vi "Valid units Read.vi"(4 "error in (no error)":errorcluster, 6 "Container State":T3, 7 "Display State In":T2) -> (0 "error out":errorcluster, 2 "Value":T1[](array[typedef]), 3 "Display State Out":T2)   [LabVIEW 2015, in "Level (G3).xctl"]
uses:
  Level (G3).xctl
  <vilib>/_xctls/Container State.ctl
  State.ctl
  Utility VIs/Controls/KRing/KRing.xctl
  Utility VIs/Controls/KNumeric (DBL)/KNumeric (DBL).xctl
  Level Units (G3).ctl
  <vilib>/_xctls/XControlSupport.lvlib
panel:
  # "Replace the Value Indicator below with an Indicator of desired type.\nDo not remove this Indicator or the others from the connector pane. \nDo not change the connector pane pattern.\nThe Value Indicator should always be the second terminal from top on the output side in the connector pane."
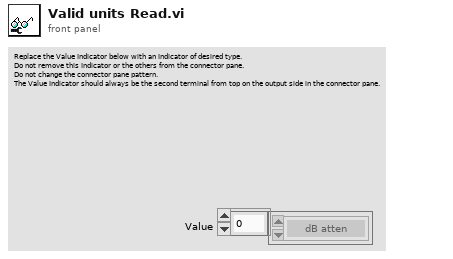
[diagram p1: front panel]
types:
  T1 = typedef "Level (G3).xctl/Level Units (G3).ctl" = enum16{"dB atten", "dB SPL", "dB re 1 Vrms", "dB V/Hz½", "dB SL", "mW", "Volts"}
  T2 = typedef "Level (G3).xctl/State.ctl" = cluster{"LMax Event":refnum<user-event>, "enable menu":bool, "Units":string[], "Valid":bool[], "multi":bool, "ctl":cluster{"Units":refnum<vi>, "Level":refnum<vi>}}
  T3 = typedef "XControlSupport.lvlib/Container State.ctl" = cluster{"Indicator?":bool, "Run Mode?":bool, " Refnum":refnum<vi>}
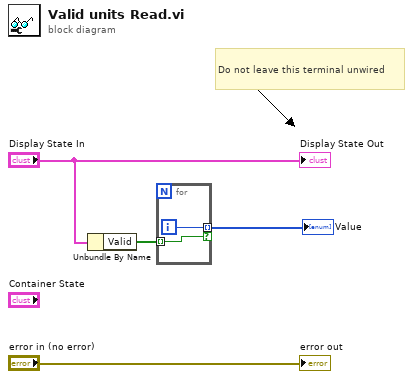
[diagram p0: block diagram]
diagram:
  # "Do not leave this terminal unwired"
  n1 = Unbundle By Name("Display State In") -> ("Valid"=w2:bool[])
  n2 = for {
    tunnel: w2 -> [w5] mode=indexing
    tunnel: [w6] -> w1 mode=indexing if=w5
    i -> [w6]
  }
  "Value" <- w1
  "error out" <- "error in (no error)"
  "Display State Out" <- "Display State In"
